vi "Initialize.vi"(8 "error in":errorcluster, 11 "Plugin in":refnum<class "PXIe-4113 DC Power Supply NI-DCPower Runtime Plugin PowerSupply.lvclass">) -> (0 "error out":errorcluster, 3 "Plugin out":refnum<class "PXIe-4113 DC Power Supply NI-DCPower Runtime Plugin PowerSupply.lvclass">)   [LabVIEW 2026, in "PXIe-4113 DC Power Supply NI-DCPower Runtime Plugin PowerSupply.lvlib" / "PXIe-4113 DC Power Supply NI-DCPower Runtime Plugin PowerSupply.lvclass"]
uses:
  PXIe-4113 DC Power Supply NI-DCPower Runtime Plugin PowerSupply.lvclass
  C:/Program Files/National Instruments/LabVIEW 2026/vi.lib/FlexLogger/SDK/PluginSDK.lvlibp/PEFClasses/SDK/Plugin/Plugin.lvclass
  <vilib>/FlexLogger/SDK/PluginSDK.lvlibp/PEFClasses/SDK/Producer Channel/Producer Channel.lvclass
  C:/Program Files/National Instruments/LabVIEW 2026/vi.lib/FlexLogger/SDK/PluginSDK.lvlibp/PEFClasses/SDK/Channel/Channel.lvclass
  <vilib>/FlexLogger/SDK/PluginSDK.lvlibp/PEFClasses/SDK/Plugin/ParameterAccess/Write String.vi
  <vilib>/FlexLogger/SDK/PluginSDK.lvlibp/PEFClasses/SDK/Plugin/ParameterAccess/Write DBL.vi
  <vilib>/FlexLogger/SDK/PluginSDK.lvlibp/PEFClasses/SDK/Producer Channel/Create Producer Channel_v2.vi
  <vilib>/FlexLogger/SDK/PluginSDK.lvlibp/PEFClasses/SDK/Plugin/Plugin.lvclass
  C:/Program Files/National Instruments/LabVIEW 2026/vi.lib/FlexLogger/SDK/PluginSDK.lvlibp/PEFClasses/SDK/Processing Element/Processing Element.lvclass
  C:/Users/krael/OneDrive - Emerson/Documents/LabVIEW Projects/FlexLogger IO Plug-ins/PXIe-4113 DC Power Supply NI-DCPower Runtime Plugin PowerSupply/PXIe-4113 DC Power Supply NI-DCPower Runtime Plugin PowerSupply.lvclass
  <vilib>/FlexLogger/SDK/PluginSDK.lvlibp
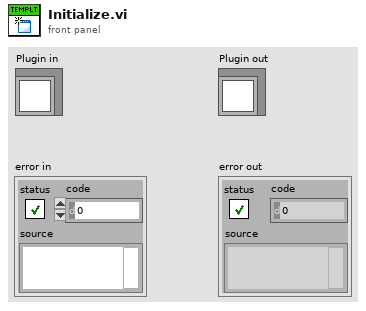
[diagram p1: front panel]
types:
  T1 = cluster{"Timing Method":enum16{"Periodic", "Immediate", "On Data Ready", "Triggered"}, "Timing Period (ms)":i32}
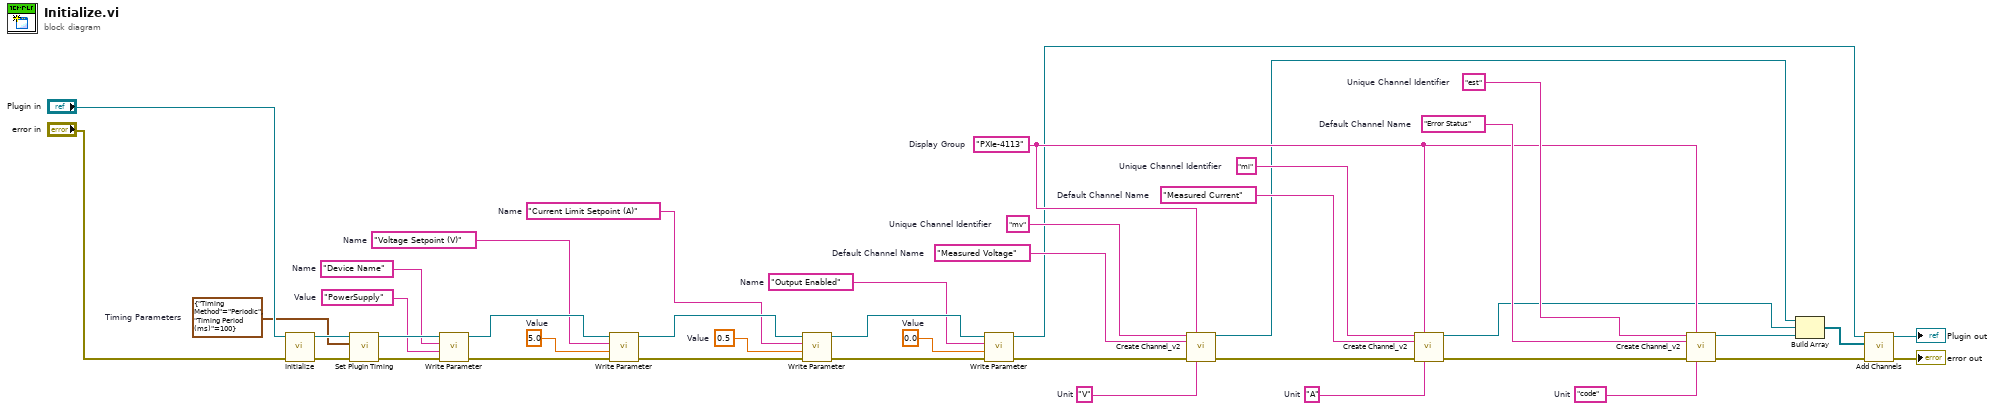
[diagram p0: block diagram]
diagram:
  w9 = "code"  # Unit
  w12 = "Error Status"  # Default Channel Name
  w13 = "est"  # Unique Channel Identifier
  w14 = "A"  # Unit
  w16 = "Measured Current"  # Default Channel Name
  w17 = "mi"  # Unique Channel Identifier
  w18 = "V"  # Unit
  w10 = "PXIe-4113"  # Display Group
  w20 = "Measured Voltage"  # Default Channel Name
  w21 = "mv"  # Unique Channel Identifier
  w23 = 0.0  # Value
  w24 = "Output Enabled"  # Name
  w27 = 0.5  # Value
  w28 = "Current Limit Setpoint (A)"  # Name
  w31 = 5.0  # Value
  w32 = "Voltage Setpoint (V)"  # Name
  w35 = "PowerSupply"  # Value
  w36 = "Device Name"  # Name
  w39 = T1 {"Timing Method"=enum."Periodic", "Timing Period (ms)"=100}  # Timing Parameters
  n1 = call-parent "Initialize.vi"("error in (no error)"="error in", "Plugin in"="Plugin in") -> ("error out"=w38:errorcluster, "Plugin out"=w40:refnum<class "PXIe-4113 DC Power Supply NI-DCPower Runtime Plugin PowerSupply.lvclass">)  [unwired: 8 in]
  n2 = call <vilib>:"Set Plugin Timing.vi"("error in (no error)"=w38, "Timing Parameters"=w39, "Plugin in"=w40) -> ("error out"=w34:errorcluster, "Plugin out"=w37:refnum<class "PXIe-4113 DC Power Supply NI-DCPower Runtime Plugin PowerSupply.lvclass">)  [unwired: 7 in]
  n3 = call-poly <vilib>:"Write Parameter.vi"("error in (no error)"=w34, "Value"=w35, "Name"=w36, "Plugin in"=w37) -> ("error out"=w30:errorcluster, "Plugin out"=w33:refnum<class "PXIe-4113 DC Power Supply NI-DCPower Runtime Plugin PowerSupply.lvclass">)  [unwired: 6 in]
  n4 = call-poly <vilib>:"Write Parameter.vi"("error in (no error)"=w30, "Value"=w31, "Name"=w32, "Plugin in"=w33) -> ("error out"=w26:errorcluster, "Plugin out"=w29:refnum<class "PXIe-4113 DC Power Supply NI-DCPower Runtime Plugin PowerSupply.lvclass">)  [unwired: 6 in]
  n5 = call-poly <vilib>:"Write Parameter.vi"("error in (no error)"=w26, "Value"=w27, "Name"=w28, "Plugin in"=w29) -> ("error out"=w22:errorcluster, "Plugin out"=w25:refnum<class "PXIe-4113 DC Power Supply NI-DCPower Runtime Plugin PowerSupply.lvclass">)  [unwired: 6 in]
  n6 = call-poly <vilib>:"Write Parameter.vi"("error in (no error)"=w22, "Value"=w23, "Name"=w24, "Plugin in"=w25) -> ("error out"=w19:errorcluster, "Plugin out"=w5:refnum<class "PXIe-4113 DC Power Supply NI-DCPower Runtime Plugin PowerSupply.lvclass">)  [unwired: 6 in]
  n7 = call-poly <vilib>:"Create Channel_v2.vi"("Unique Channel Identifier"=w21, "Display Group"=w10, "Default Channel Name"=w20, "error in (no error)"=w19, "Unit"=w18) -> ("Producer Channel"=w8:refnum<class "Producer Channel.lvclass">, "error out"=w15:errorcluster)  [unwired: 9 in]
  n8 = call-poly <vilib>:"Create Channel_v2.vi"("Unique Channel Identifier"=w17, "Display Group"=w10, "Default Channel Name"=w16, "error in (no error)"=w15, "Unit"=w14) -> ("Producer Channel"=w7:refnum<class "Producer Channel.lvclass">, "error out"=w11:errorcluster)  [unwired: 9 in]
  n9 = call-poly <vilib>:"Create Channel_v2.vi"("Unique Channel Identifier"=w13, "Display Group"=w10, "Default Channel Name"=w12, "error in (no error)"=w11, "Unit"=w9) -> ("Producer Channel"=w6:refnum<class "Producer Channel.lvclass">, "error out"=w3:errorcluster)  [unwired: 9 in]
  n10 = Build Array(w8, w7, w6) -> (w4:refnum<class "Producer Channel.lvclass">[])
  n11 = call <vilib>:"Add Channels.vi"("error in (no error)"=w3, "Channels"=w4, "Plugin in"=w5) -> ("error out"=→"error out":errorcluster, "Plugin out"=→"Plugin out":refnum<class "PXIe-4113 DC Power Supply NI-DCPower Runtime Plugin PowerSupply.lvclass">)  [unwired: 7 in]
